vi "Initialize.vi"(8 "error in (no error)":errorcluster, 10 "Path Command Text":string, 11 "PathTokenizer in":refnum<class "PathTokenizer.lvclass">) -> (0 "error out":errorcluster, 3 "PathTokenizer out":refnum<class "PathTokenizer.lvclass">)   [LabVIEW 2019, in "PathTokenizer.lvclass"]
uses:
  PathTokenizer.lvclass
  PathTokenizer.lvclass/PathTokenizer.ctl
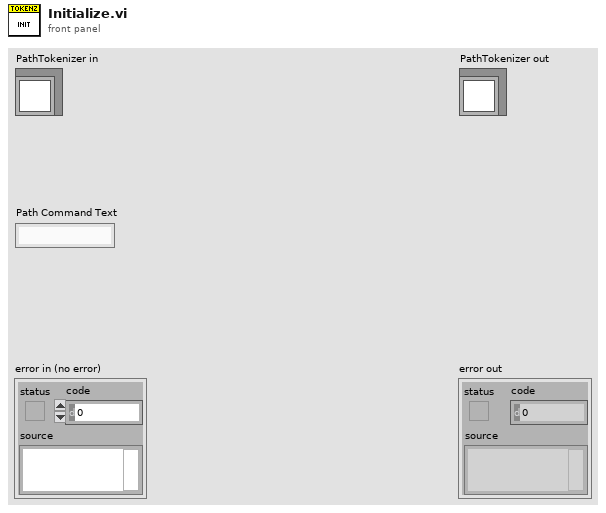
[diagram p1: front panel]
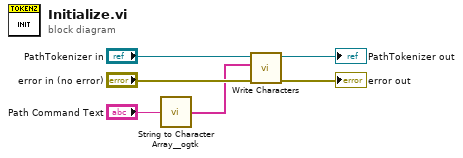
[diagram p0: block diagram]
diagram:
  n1 = call <userlib>:"String to Character Array__ogtk.vi"("Input String"="Path Command Text") -> ("Character Array"=w1:string[])
  n2 = call "Write Characters.vi"("error in (no error)"="error in (no error)", "Characters"=w1, "PathTokenizer in"="PathTokenizer in") -> ("error out"=→"error out":errorcluster, "PathTokenizer out"=→"PathTokenizer out":refnum<class "PathTokenizer.lvclass">)  [unwired: 7 in]
